vi "Dispose.vi"(8 "error in (no error)":errorcluster, 11 "EventsParent in":refnum<class "Events.lvclass">) -> (0 "error out":errorcluster, 3 "EventsParent out":refnum<class "Events.lvclass">)   [LabVIEW 2020, in "wamplv.lvlib" / "Events.lvclass"]
uses:
  Events.lvclass
  Events.lvclass/Events.ctl
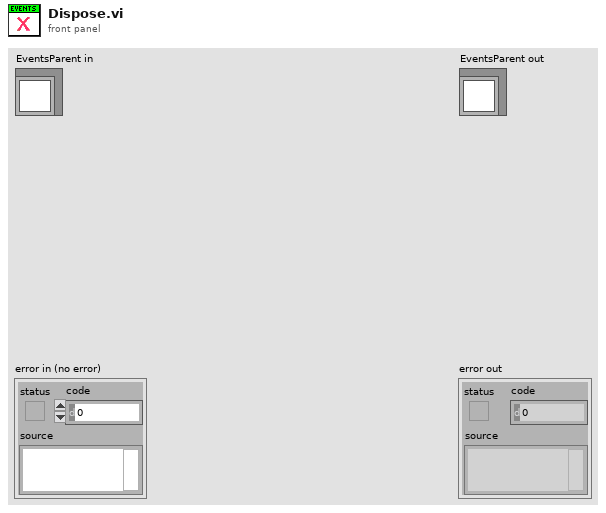
[diagram p1: front panel]
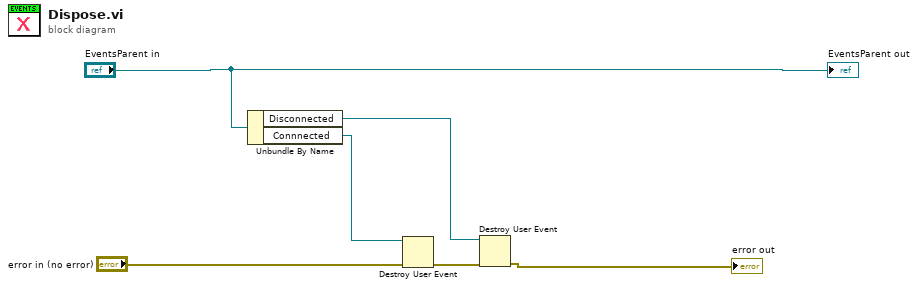
[diagram p0: block diagram]
diagram:
  n1 = Unbundle By Name("EventsParent in") -> ("Disconnected"=w3:refnum<user-event>, "Connnected"=w1:refnum<user-event>)
  n2 = Destroy User Event(user event=w1, error in="error in (no error)") -> (error out=w2:errorcluster)
  n3 = Destroy User Event(user event=w3, error in=w2) -> (error out=→"error out":errorcluster)
  "EventsParent out" <- "EventsParent in"
